vi "CheckSum_8bit.vi"(11 "字符串":string) -> (3 "和":u32 format="%x")   [LabVIEW 2018]
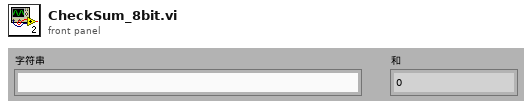
[diagram p1: front panel]
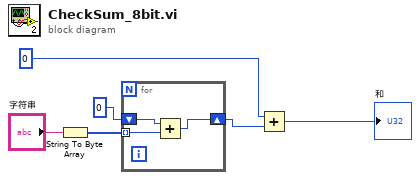
[diagram p0: block diagram]
diagram:
  n1 = String To Byte Array(string="字符串") -> (unsigned byte array=w4:u8[])
  n2 = for {
    tunnel: w4 -> [w8] mode=indexing
    shift-right: [w7] -> w2
    shift-left: u8 0 ("和") -> [w9]
    n3 = Add(x=w9, y=w8) -> (x+y=w7:u8)
  }
  n4 = Add(x=u8 0 ("和"), y=w2) -> (x+y=→"和":u8)
